vi "HDI Bond Pad TR Match.vi"(9 "error in (no error)":errorcluster, 10 "Image Src":T1) -> (0 "error out":errorcluster, 1 "In Range?":bool, 2 "y rel move":dbl, 3 "x rel move":dbl, 4 "Vertical vector":dbl[](array[numeric]), 5 "Angle Between Lines":dbl)   [LabVIEW 2011]
uses:
  <vilib>/vision/Image Controls.llb/IMAQ Image.ctl
  <vilib>/vision/NI_Vision_Development_Module.lvlib
  <vilib>/vision/driver/NI_Vision_Acquisition_Software.lvlib
panel:
  in  "Scale Factor":sgl=0.000429
  out "y":sgl
  out "x":sgl
  out "X Coordinate Pixels":dbl
  out "Y Coordinate Pixels":sgl
  out "Remaining Outputs":T2 {"Horizontal calibrated"."Point2"."Y" format="%.2f"; "Horizontal calibrated"."Point2"."X" format="%.2f"; "Horizontal calibrated"."Point1"."Y" format="%.2f"; "Horizontal calibrated"."Point1"."X" format="%.2f"; "Horizontal"."Point2"."Y" format="%.2f"; "Horizontal"."Point2"."X" format="%.2f"; "Horizontal"."Point1"."Y" format="%.2f"; "Horizontal"."Point1"."X" format="%.2f"; "Edge Coordinates (calibrated) (Straight Edge (Rake) 2)"."Y" format="%.2f"; "Edge Coordinates (calibrated) (Straight Edge (Rake) 2)"."X" format="%.2f"; "Edge Coordinates (Straight Edge (Rake) 2)"."Y" format="%.2f"; "Edge Coordinates (Straight Edge (Rake) 2)"."X" format="%.2f"}
  out "Vertical Calibrated":T3 {"Point2"."Y" format="%.2f"; "Point2"."X" format="%.2f"; "Point1"."Y" format="%.2f"; "Point1"."X" format="%.2f"}
  out "Hori":cluster{"X":sgl, "Y":sgl}[](array[cluster]) {"Y" format="%.2f"; "X" format="%.2f"}
  out "Vertical rake":T3 {"Point2"."Y" format="%.2f"; "Point2"."X" format="%.2f"; "Point1"."Y" format="%.2f"; "Point1"."X" format="%.2f"}
  out "Edge Coordinates (Straight Edge (Rake) 1)":cluster{"X":sgl, "Y":sgl}[](array[cluster]) {"Y" format="%.2f"; "X" format="%.2f"}
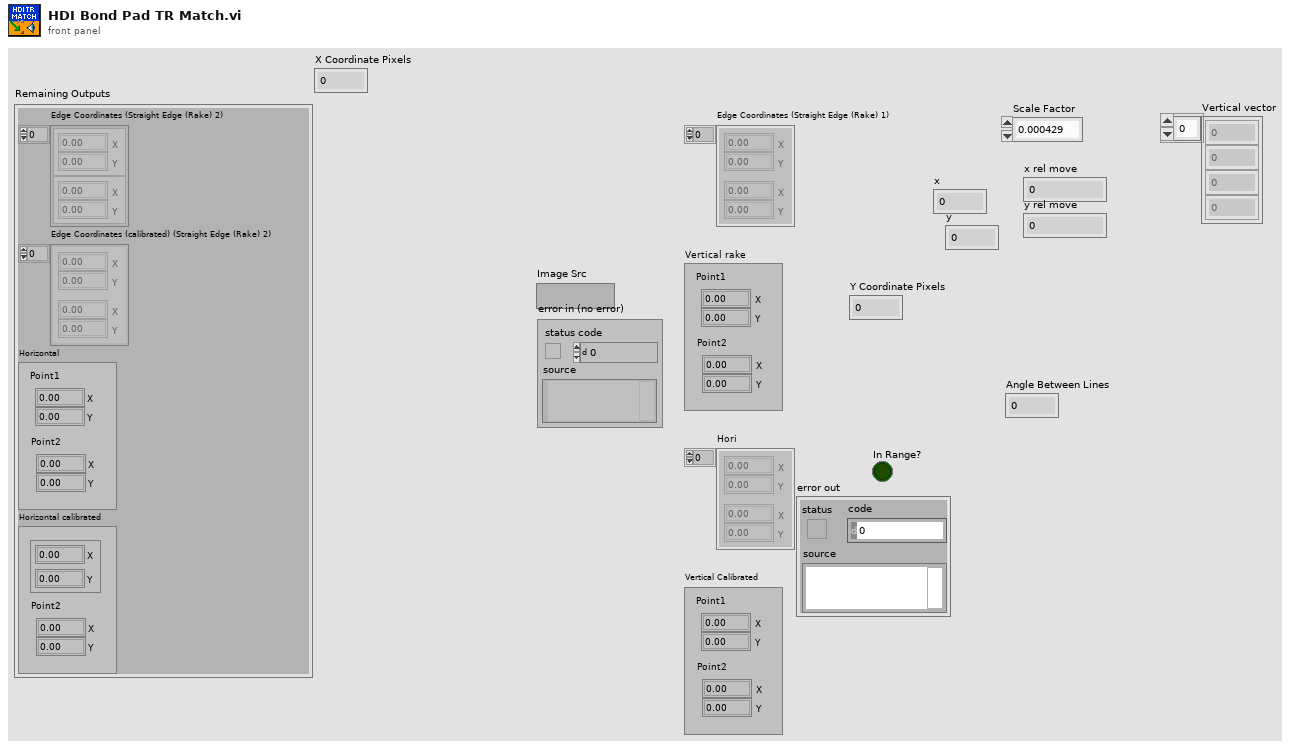
[diagram p1: front panel]
types:
  T1 = typedef "IMAQ Image.ctl" = refnum<image>
  T2 = cluster{"Edge Coordinates (Straight Edge (Rake) 2)":cluster{"X":sgl, "Y":sgl}[], "Edge Coordinates (calibrated) (Straight Edge (Rake) 2)":cluster{"X":sgl, "Y":sgl}[], "Horizontal":cluster{"Point1":cluster{"X":sgl, "Y":sgl}, "Point2":cluster{"X":sgl, "Y":sgl}}, "Horizontal calibrated":cluster{"Point1":cluster{"X":sgl, "Y":sgl}, "Point2":cluster{"X":sgl, "Y":sgl}}}
  T3 = cluster{"Point1":cluster{"X":sgl, "Y":sgl}, "Point2":cluster{"X":sgl, "Y":sgl}}
  T4 = cluster{"Global Rectangle":i32[], "Contours":cluster{"ID":enum32{"External", "Internal"}, "Type":u32, "Coordinates":i32[]}[]}
  T5 = cluster{"Contrast":i32, "Filter width":i32, "Steepness":i32, "Subsampling Ratio":u32, "Scan Direction":u32, "Show Search Area":bool, "Show Search Lines":bool, "Show Edges Found":bool, "Show Result":bool}
  T6 = typedef "IMAQdx.ctl" = refnum<k21>
  T7 = typedef "IMAQ Rectangle" = cluster{"Left":i32, "Top":i32, "Right":i32, "Bottom":i32, "Rotation":dbl}
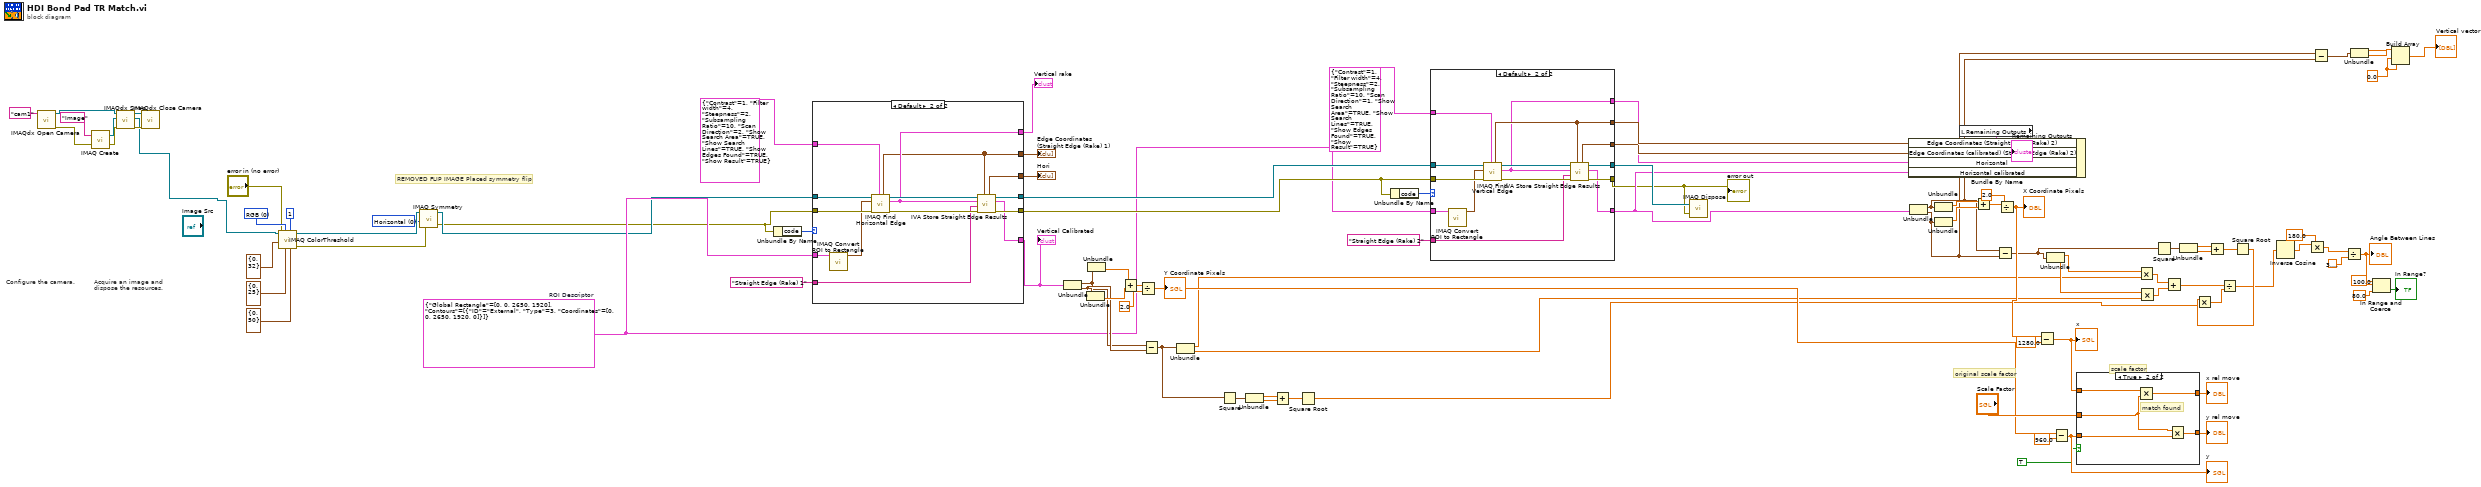
[diagram p0: block diagram]
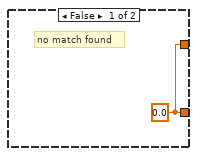
[diagram p2: hidden frame]
diagram:
  w10 = u32 0 items=["Horizontal", "Vertical", "Central", "1st Diagonal", "2nd Diagonal"] ("Type of Symmetry")
  w15 = T4 {"Global Rectangle"=[0, 0, 2650, 1920], "Contours"=[{"ID"=enum."External", "Type"=3, "Coordinates"=[0, 0, 2650, 1920, 0]}]}  # ROI Descriptor
  w22 = 0.0
  w96 = u16 0 items=["RGB", "HSL", "HSV", "HSI"] ("Color Mode")
  # "REMOVED FLIP IMAGE Placed symmetry flip"
  # "original scale factor"
  # "scale factor"
  # "Acquire an image and\ndispose the resources."
  # "Configure the camera."
  n1 = call <vilib>:"IMAQdx Open Camera.vi"("Session In"="cam1" ("Interface Name")) -> ("error out"=w4:errorcluster, "Session Out"=w9:T6)  [unwired: 9 in]
  n2 = call "IMAQ Create"("Image Name"="Image", "error in (no error)"=w4) -> ("New Image"=w7:T1, "error out"=w8:errorcluster)  [unwired: 3 in]
  n3 = call <vilib>:"IMAQdx Snap.vi"("error in"=w8, "Image In"=w7, "Session In"=w9) -> ("error out"=w6:errorcluster, "Image Out"=w1:T1, "Session Out"=w5:T6)  [unwired: 6 in]
  n4 = call <vilib>:"IMAQdx Close Camera.vi"("error in"=w6, "Session In"=w5) -> ()  [unwired: 9 in, 1 out]
  n5 = call "IMAQ ColorThreshold"("Blue or Luma or Val or Inten Range"=cluster{"Lower value":i32, "Upper value":i32} {"Lower value"=0, "Upper value"=50}, "Replace Value"=1, "Green or Sat Range"=cluster{"Lower value":i32, "Upper value":i32} {"Lower value"=0, "Upper value"=25}, "Color Mode"=w96, "error in (no error)"="error in (no error)", "Red or Hue Range"=cluster{"Lower value":i32, "Upper value":i32} {"Lower value"=0, "Upper value"=32}, "Image Src"=w1) -> ("error out"=w12:errorcluster, "Image Dst Out"=w14:T1)  [unwired: 3 in]
  n6 = call "IMAQ Symmetry"("error in (no error)"=w12, "Type of Symmetry"=w10, "Image Src"=w14) -> ("error out"=w11:errorcluster, "Image Dst Out"=w13:T1)  [unwired: 2 in]
  n7 = Unbundle By Name(w11) -> ("code"=w86:i32)
  n8 = case shown="Default" w86 {
    tunnel: T5 {"Contrast"=1, "Filter width"=4, "Steepness"=2, "Subsampling Ratio"=10, "Scan Direction"=2, "Show Search Area"=TRUE, "Show Search Lines"=TRUE, "Show Edges Found"=TRUE, "Show Result"=TRUE} ("Settings (Straight Edge (Rake) 1)") -> [_ w112]
    tunnel: w13 -> [w98 w111]
    tunnel: w11 -> [_ w110]
    tunnel: w15 -> [_ w109]
    tunnel: [w98 w106] -> w85
    tunnel: [_ w104] -> w91
    tunnel: [_ w103] -> w90
    tunnel: [_ w102] -> w89
    tunnel: "Straight Edge (Rake) 1" ("Step Name") -> [_ w101]
    tunnel: [_ w100] -> w87
    tunnel: [_ w99] -> w75
    frame -1074396199, -1074396198 {
      # "Discard Coordinate System Error"
    }
    frame Default {
      n9 = call "IMAQ Convert ROI to Rectangle"("ROI Descriptor"=w109) -> ("Rectangle"=w108:T7)  [unwired: 8 in, 1 out]
      n10 = call "IMAQ Find Horizontal Edge"("Settings"=w112, "error in (no error)"=w110, "Rectangle"=w108, "Image"=w111) -> ("error out"=w105:errorcluster, "Line Coordinates"=w103:T3, "Image Out"=w107:T1, "Edge Coordinates"=w102:cluster{"X":sgl, "Y":sgl}[])  [unwired: 2 in, 2 out]
      n11 = call <vilib>:"IVA Store Straight Edge Results.vi"("Edge Coordinates"=w102, "error in (no error)"=w105, "Step Name"=w101, "Line Coordinates"=w103, "Image in"=w107) -> ("error out"=w104:errorcluster, "Line Coordinates (calibrated)"=w99:T3, "Image dup"=w106:T1, "Edge Coordinates (calibrated)"=w100:cluster{"X":sgl, "Y":sgl}[])  [unwired: 3 in]
    }
  }
  "Edge Coordinates (Straight Edge (Rake) 1)" <- w89
  "Vertical rake" <- w90
  "Hori" <- w87
  "Vertical Calibrated" <- w75
  n12 = Unbundle(w75) -> ("Point1"=w23:cluster{"X":sgl, "Y":sgl}, "Point2"=w24:cluster{"X":sgl, "Y":sgl})
  n13 = Unbundle(w24) -> ("Y"=w73:sgl)  [unwired: 1 out]
  n14 = Unbundle(w23) -> ("Y"=w74:sgl)  [unwired: 1 out]
  n15 = Add(x=w74, y=w73) -> (x+y=w72:sgl)
  n16 = Divide(x=w72, y=sgl 2.0) -> (x/y=w58:sgl)
  "Y Coordinate Pixels" <- w58
  n17 = Subtract(x=w23, y=w24) -> (x-y=w40:cluster{"X":sgl, "Y":sgl})
  n18 = Unbundle(w40) -> ("X"=w53:sgl, "Y"=w52:sgl)
  n19 = Square(x=w40) -> (x^2=w44:cluster{"X":sgl, "Y":sgl})
  n20 = Unbundle(w44) -> ("X"=w43:sgl, "Y"=w42:sgl)
  n21 = Add(x=w43, y=w42) -> (x+y=w41:sgl)
  n22 = Square Root(x=w41) -> (sqrt(x)=w37:sgl)
  n23 = Unbundle By Name(w91) -> ("code"=w79:i32)
  n24 = case shown="Default" w79 {
    tunnel: w85 -> [w113 w127]
    tunnel: w91 -> [_ w126]
    tunnel: T5 {"Contrast"=1, "Filter width"=4, "Steepness"=2, "Subsampling Ratio"=10, "Scan Direction"=1, "Show Search Area"=TRUE, "Show Search Lines"=TRUE, "Show Edges Found"=TRUE, "Show Result"=TRUE} ("Settings (Straight Edge (Rake) 2)") -> [_ w125]
    tunnel: w15 -> [_ w124]
    tunnel: [w113 w121] -> w78
    tunnel: [_ w119] -> w25
    tunnel: [_ w118] -> w83
    tunnel: [_ w117] -> w82
    tunnel: [_ w116] -> w70
    tunnel: [_ w115] -> w81
    tunnel: "Straight Edge (Rake) 2" ("Step Name") -> [_ w114]
    frame -1074396199, -1074396198 {
      # "Discard Coordinate System Error"
    }
    frame Default {
      n25 = call "IMAQ Convert ROI to Rectangle"("ROI Descriptor"=w124) -> ("Rectangle"=w123:T7)  [unwired: 8 in, 1 out]
      n26 = call "IMAQ Find Vertical Edge"("Settings"=w125, "error in (no error)"=w126, "Rectangle"=w123, "Image"=w127) -> ("error out"=w120:errorcluster, "Line Coordinates"=w115:T3, "Image Out"=w122:T1, "Edge Coordinates"=w118:cluster{"X":sgl, "Y":sgl}[])  [unwired: 2 in, 2 out]
      n27 = call <vilib>:"IVA Store Straight Edge Results.vi"("Edge Coordinates"=w118, "error in (no error)"=w120, "Step Name"=w114, "Line Coordinates"=w115, "Image in"=w122) -> ("error out"=w119:errorcluster, "Line Coordinates (calibrated)"=w116:T3, "Image dup"=w121:T1, "Edge Coordinates (calibrated)"=w117:cluster{"X":sgl, "Y":sgl}[])  [unwired: 3 in]
    }
  }
  "error out" <- w25
  n28 = call "IMAQ Dispose"("Image"=w78, "error in (no error)"=w25) -> ()  [unwired: 4 in, 1 out]
  n29 = Unbundle(w70) -> ("Point1"=w20:cluster{"X":sgl, "Y":sgl}, "Point2"=w19:cluster{"X":sgl, "Y":sgl})
  n30 = Unbundle(w20) -> ("X"=w67:sgl)  [unwired: 1 out]
  n31 = Unbundle(w19) -> ("X"=w66:sgl)  [unwired: 1 out]
  n32 = local read "Remaining Outputs"() -> (w76:T2)
  n33 = Bundle By Name(cluster=w76, "Edge Coordinates (Straight Edge (Rake) 2)"=w83, "Edge Coordinates (calibrated) (Straight Edge (Rake) 2)"=w82, "Horizontal"=w81, "Horizontal calibrated"=w70) -> (→"Remaining Outputs":T2)
  n34 = Add(x=w67, y=w66) -> (x+y=w69:sgl)
  n35 = Subtract(x=w20, y=w19) -> (x-y=w49:cluster{"X":sgl, "Y":sgl})
  n36 = Divide(x=w69, y=2.0) -> (x/y=w57:dbl)
  "X Coordinate Pixels" <- w57
  n37 = Subtract(x=w57, y=sgl 1280.0) -> (x-y=w62:dbl)
  "x" <- w62
  n38 = Unbundle(w49) -> ("X"=w55:sgl, "Y"=w54:sgl)
  n39 = Subtract(x=w58, y=sgl 960.0) -> (x-y=w63:sgl)
  "y" <- w63
  n40 = case shown="True" TRUE {
    tunnel: w63 -> [_ w133]
    tunnel: w62 -> [_ w132]
    tunnel: [w128 w131] -> w61
    tunnel: [w128 w130] -> w60
    tunnel: "Scale Factor" -> [_ w129]
    frame False {
      w128 = sgl 0.0
      # "no match found"
    }
    frame True {
      # "match found"
      n41 = Multiply(x=w132, y=w129) -> (x*y=w131:dbl)
      n42 = Multiply(x=w129, y=w133) -> (x*y=w130:sgl)
    }
  }
  "x rel move" <- w61
  "y rel move" <- w60
  n43 = Multiply(x=w55, y=w53) -> (x*y=w51:sgl)
  n44 = Multiply(x=w54, y=w52) -> (x*y=w50:sgl)
  n45 = Square(x=w49) -> (x^2=w48:cluster{"X":sgl, "Y":sgl})
  n46 = Add(x=w51, y=w50) -> (x+y=w39:sgl)
  n47 = Unbundle(w48) -> ("X"=w47:sgl, "Y"=w46:sgl)
  n48 = Add(x=w47, y=w46) -> (x+y=w45:sgl)
  n49 = Square Root(x=w45) -> (sqrt(x)=w38:sgl)
  n50 = Multiply(x=w38, y=w37) -> (x*y=w36:sgl)
  n51 = Divide(x=w39, y=w36) -> (x/y=w35:sgl)
  n52 = Inverse Cosine(1:w35) -> (0:w34:sgl)
  n53 = Multiply(x=w34, y=sgl 180.0) -> (x*y=w32:sgl)
  n54 = Subtract(x=w19, y=w20) -> (x-y=w18:cluster{"X":sgl, "Y":sgl})
  n55 = Divide(x=w32, y=3.141592653589793) -> (x/y=w30:dbl)
  "Angle Between Lines" <- w30
  n56 = Unbundle(w18) -> ("X"=w16:sgl, "Y"=w17:sgl)
  n57 = In Range and Coerce(upper limit=100.0, x=w30, lower limit=80.0) -> (In Range?=→"In Range?":bool)  [unwired: 1 out]
  n58 = Build Array(w17, w16, w22, w22) -> (→"Vertical vector":dbl[])
